vi "Config Pulse I Measure V.vi"(0 "VISA resource name":refnum<visa-resource-name>, 1 "Channel (Channel A)":T1, 2 "On Time":dbl=0.001, 3 "Off Time":dbl=0.001, 4 "Points (1)":u32=1 min=1, 5 "error in":errorcluster, 6 "Bias (0)":dbl, 7 "Sync In":u32, 8 "Level":dbl=0.001, 9 "Sync Out":u32, 10 "Limit":dbl=1.0, 11 "Sync In Timeout (10e-3)":dbl, 12 "Tag (1)":u32=1 min=1, 15 "Sync In Abort (True)":bool=TRUE) -> (13 "Command String":string, 14 "VISA resource name out":refnum<visa-resource-name>, 17 "Success":bool, 18 "Message":string, 19 "error out":errorcluster)   [LabVIEW 2018, in "Keithley 2600 Series.lvlib"]
doc: "This VI configures a current pulse train using the KIFactoryPulse script.\n\n<b>Functions and Attributes Used</b>\nConfigPulseIMeasureV()"
uses:
  Keithley 2600 Series.lvlib
  Private/GlobalVariables.vi
  Channel.ctl
panel:
  in  "Buffer (nil)":string="nil"
  # "(c) 2008 Keithley Instruments, Inc.  ALL RIGHTS RESERVED."
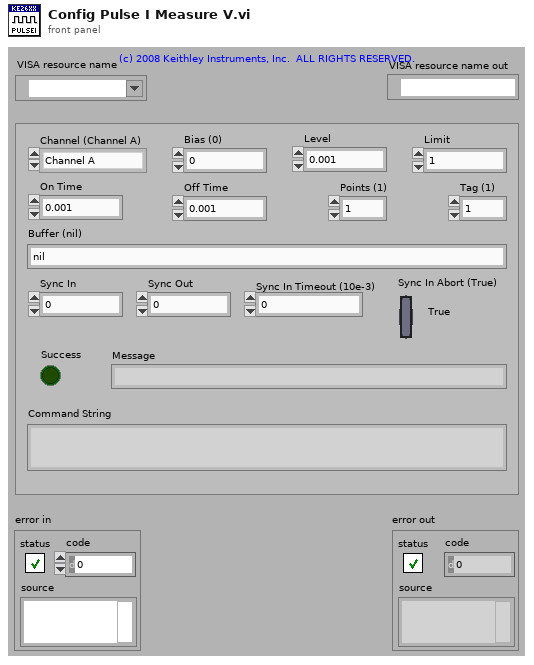
[diagram p1: front panel]
types:
  T1 = typedef "Keithley 2600 Series.lvlib/Channel.ctl" = enum32{"Channel A", "Channel B"}
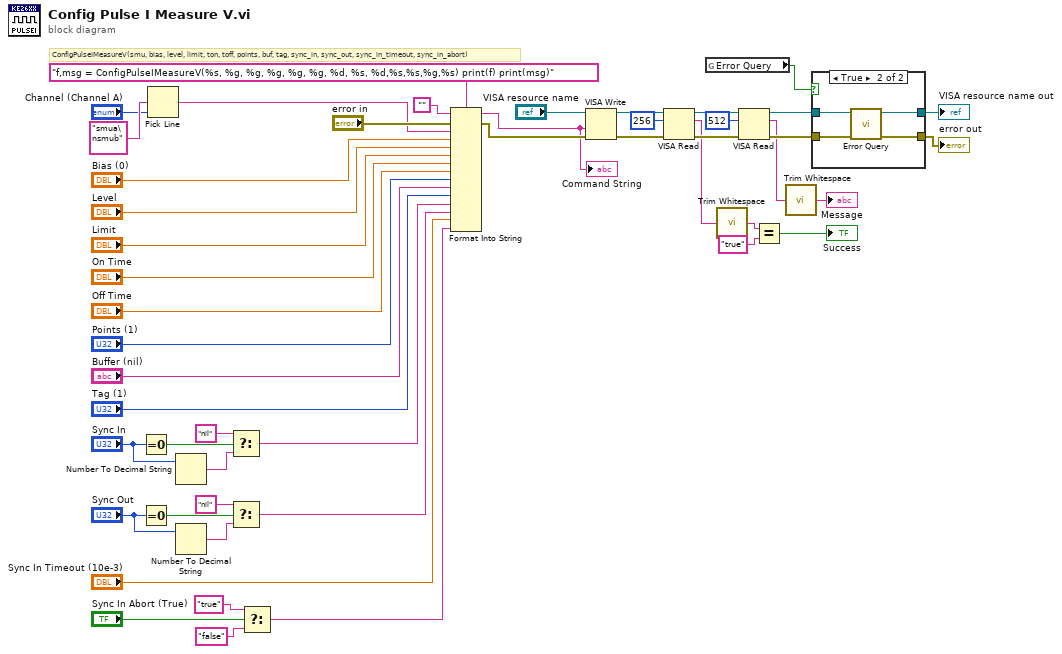
[diagram p0: block diagram]
diagram:
  # "ConfigPulseIMeasureV(smu, bias, level, limit, ton, toff, points, buf, tag, sync_in, sync_out, sync_in_timeout, sync_in_abort)"
  n1 = Equal To 0?(x="Sync In") -> (x = 0?=w35:bool)
  n2 = Equal To 0?(x="Sync Out") -> (x = 0?=w31:bool)
  n3 = Pick Line(multi-line string="smua\nsmub", line index="Channel (Channel A)") -> (output string=w44:string)  [unwired: 1 out]
  n4 = Number To Decimal String(number="Sync In") -> (decimal integer string=w32:string)  [unwired: 1 out]
  n5 = Number To Decimal String(number="Sync Out") -> (decimal integer string=w29:string)  [unwired: 1 out]
  n6 = Select(t="nil", s=w35, f=w32) -> (s? t:f=w24:string)
  n7 = Select(t="nil", s=w31, f=w29) -> (s? t:f=w23:string)
  n8 = Select(t="true", s="Sync In Abort (True)", f="false") -> (s? t:f=w21:string)
  n9 = Format Into String(format string="f,msg = ConfigPulseIMeasureV(%s, %g, %g, %g, %g, %g, %d, %s, %d,%s,%s,%g,%s) print(f) print(msg)", initial string="", error in="error in", w44, "Bias (0)", "Level", "Limit", "On Time", "Off Time", "Points (1)", "Buffer (nil)", "Tag (1)", w24, w23, "Sync In Timeout (10e-3)", w21) -> (resulting string=w6:string, error out=w20:errorcluster)
  "Command String" <- w6
  n10 = VISA Write(VISA resource name="VISA resource name", write buffer=w6, error in (no error)=w20) -> (VISA resource name out=w17:refnum<visa-resource-name>, error out=w18:errorcluster)  [unwired: 1 out]
  n11 = VISA Read(VISA resource name=w17, byte count=u32 256, error in (no error)=w18) -> (VISA resource name out=w16:refnum<visa-resource-name>, read buffer=w14:string, error out=w15:errorcluster)  [unwired: 1 out]
  n12 = global read "GlobalVariables.vi" "Error Query"() -> (w10:bool)
  n13 = call <vilib>:"Trim Whitespace.vi"("string"=w14) -> ("trimmed string"=w13:string)  [unwired: 1 in]
  n14 = VISA Read(VISA resource name=w16, byte count=u32 512, error in (no error)=w15) -> (VISA resource name out=w8:refnum<visa-resource-name>, read buffer=w1:string, error out=w9:errorcluster)  [unwired: 1 out]
  n15 = Equal?(x=w13, y="true") -> (x = y?=→"Success":bool)
  n16 = call <vilib>:"Trim Whitespace.vi"("string"=w1) -> ("trimmed string"=→"Message":string)  [unwired: 1 in]
  n17 = case shown="True" w10 {
    tunnel: w8 -> [w51 w55]
    tunnel: w9 -> [w50 w54]
    tunnel: [w51 w53] -> w7
    tunnel: [w50 w52] -> w5
    frame False {
    }
    frame True {
      n18 = call "Error Query.vi"("error in (no error)"=w54, "VISA resource name"=w55) -> ("error out"=w52:errorcluster, "VISA resource name out"=w53:refnum<visa-resource-name>)  [unwired: 8 out]
    }
  }
  "VISA resource name out" <- w7
  "error out" <- w5
